vi "多参数断电保存全局变量.vi"() -> ()   [LabVIEW 2022 SP3, in "斯坦道原位多参数.lvlib"]
panel:
  in  "电导率单位":enum16{"mS/cm", "μS/cm"}(ring)
  in  "第三点信号值":sgl
  in  "第三点检测值":sgl
  in  "第三点标准值":sgl
  in  "第二点信号值":sgl
  in  "第二点检测值":sgl
  in  "第二点标准值":sgl
  in  "第一点信号值":sgl
  in  "第一点检测值":sgl
  in  "第一点标准值":sgl
  in  "校准类型":u16(ring) caption="校准类型：" items=["单点校准"=1, "两点校准"=2, "三点校准"=3]
  out "校准时间":timestamp caption="校准时间：" format="%<%x %X>T"
  in  "传感器类型":enum16{"STD自研", "纳清"}(ring)
  in  "波特率":u32(ring)=115200 items=["9600"=9600, "19200"=19200, "115200"=115200]
  in  "传感器参数自动获取":bool=TRUE
  out "传感器参数modbus":u16[](array[numeric])
  in  "标样测试组数":dbl=1.0 caption="标样测试组数:"
  in  "水样测试组数":dbl=1.0 caption="水样测试组数:"
  in  "转刷清洗时间":dbl=30.0 caption="转刷清洗时间:"
  in  "上电初始化时间":dbl=5.0 caption="上电初始化时间:"
  in  "水样稳定时间":dbl=5.0 caption="水样稳定时间:"
  in  "VISA Resource":refnum<visa-resource-name>="COM6"
  in  "运行周期":T1
  in  "质控参数设置":T2
  # "组"
  # "min"
  # "组"
  # "s"
  # "s"
  # "运行模式："
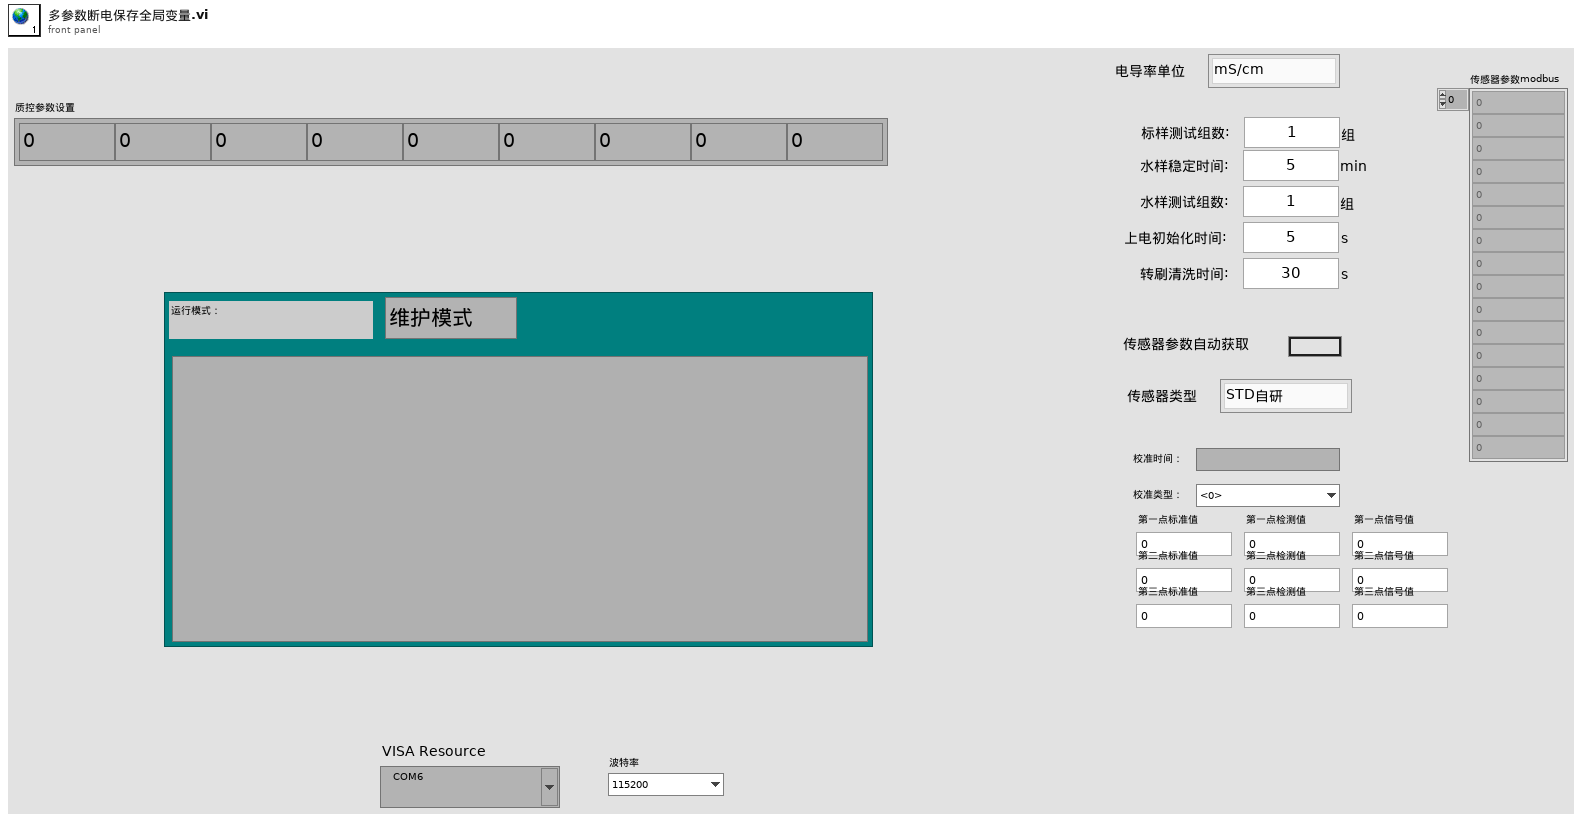
[diagram p1: front panel]
types:
  T1 = cluster{"运行模式":enum16{"维护模式", "常规模式", "应急模式", "质控模式"}, "24H周期设置":bool[]}
  T2 = cluster{"水温标准液标准浓度":dbl, "酸碱度标准液标准浓度":dbl, "溶解氧标准液标准浓度":dbl, "电导率标准液标准浓度":dbl, "浊度标准液标准浓度":dbl, "叶绿素a标准液标准浓度":dbl, "蓝绿藻标准液标准浓度":dbl, "ORP标准液标准浓度":dbl, "藻密度标准液标准浓度":dbl}
diagram:
